vi "Update SBlockk.vi"(8 "error in (no error)":errorcluster, 9 "element":refnum<class "Schedule Block.lvclass">, 10 "Index":i32, 11 "Sequence of SBlocks in":refnum<class "Sequence of SBlocks.lvclass">) -> (0 "error out":errorcluster, 3 "Sequence of SBlocks out":refnum<class "Sequence of SBlocks.lvclass">)   [LabVIEW 2020, in "CIRCUS_uServices.lvlib" / "Run Utilities.lvlib" / "Sequence of SBlocks.lvclass"]
uses:
  Sequence of SBlocks.lvclass
  Sequence of SBlocks.lvclass/Sequence of SBlocks.ctl
  Schedule Block/Schedule Block.lvclass
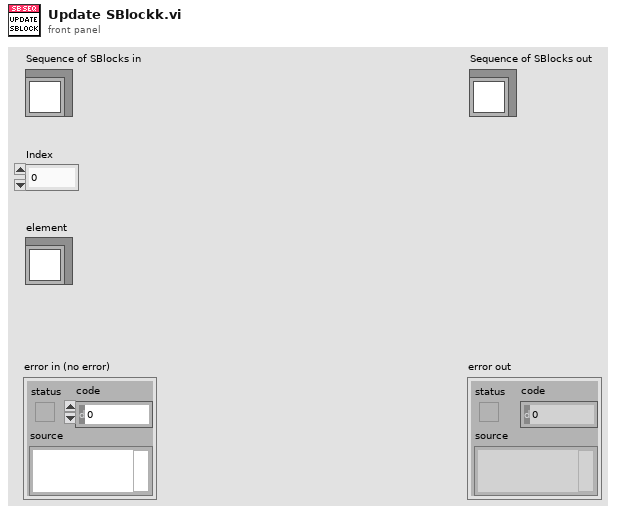
[diagram p1: front panel]
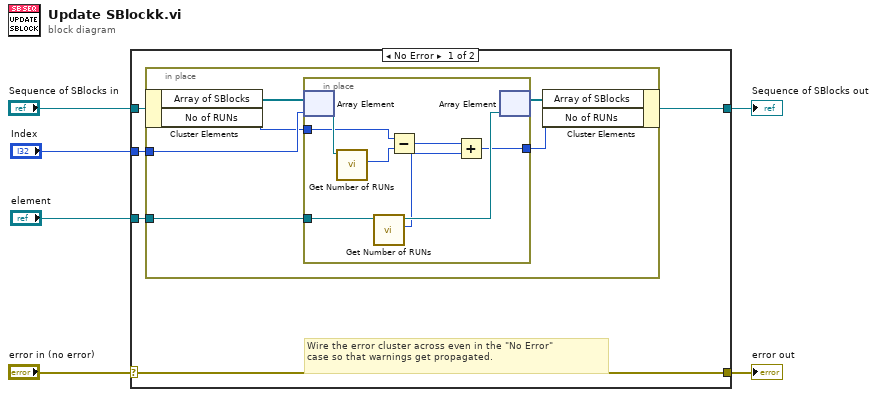
[diagram p0: block diagram]
diagram:
  n1 = case shown="No Error" "error in (no error)" {
    selector: "error in (no error)" -> [w11 w27]
    tunnel: [w11 w27] -> w5
    tunnel: [w7 w26] -> w3
    tunnel: "Sequence of SBlocks in" -> [w10 w26]
    tunnel: "Index" -> [w9 _]
    tunnel: "element" -> [w8 _]
    frame No Error {
      # "Wire the error cluster across even in the \"No Error\"\ncase so that warnings get propagated."
      n2 = in-place {
        in-place-border: w9 -> [w16]
        in-place-border: w8 -> [w15]
        n3 = in-place-cluster #1(w10) -> ("Array of SBlocks"=w17:refnum<class "Schedule Block.lvclass">[], "No of RUNs"=w13:i32)
        n4 = in-place {
          in-place-border: w15 -> [w22]
          in-place-border: w13 -> [w24]
          in-place-border: [w18] -> w12
          n5 = in-place-array #2(w17, w16) -> (w25:refnum<class "Schedule Block.lvclass">)
          n6 = call-dynamic "Get Number of RUNs.vi"("Schedule Block in"=w25) -> ("No. of RUNs"=w23:i32)  [unwired: 8 in, 2 out]
          n7 = call-dynamic "Get Number of RUNs.vi"("Schedule Block in"=w22) -> ("No. of RUNs"=w19:i32, "Schedule Block out"=w21:refnum<class "Schedule Block.lvclass">)  [unwired: 8 in, 1 out]
          n8 = Subtract(x=w24, y=w23) -> (x-y=w20:i32)
          n9 = Add(x=w20, y=w19) -> (x+y=w18:i32)
          n10 = in-place-array #2(w21) -> (w14:refnum<class "Schedule Block.lvclass">[])  [unwired: 1 out]
        }
        n11 = in-place-cluster #1("Array of SBlocks"=w14, "No of RUNs"=w12) -> (w7:refnum<class "Sequence of SBlocks.lvclass">)
      }
    }
    frame Error {
    }
  }
  "error out" <- w5
  "Sequence of SBlocks out" <- w3
